vi "edittest handle delete sequence.vi"(6 "User Information":T2, 8 "error in (no error)":errorcluster, 10 "Test Sequence Id (\"\")":string, 11 "Connection Refnum":T1) -> (0 "error out":errorcluster, 3 "Connection Refnum":T1)   [LabVIEW 2011]
uses:
  server/database/Users/User Record.ctl
  Summitek EXT/ODBC/SQL Controls/Connection Refnum.ctl
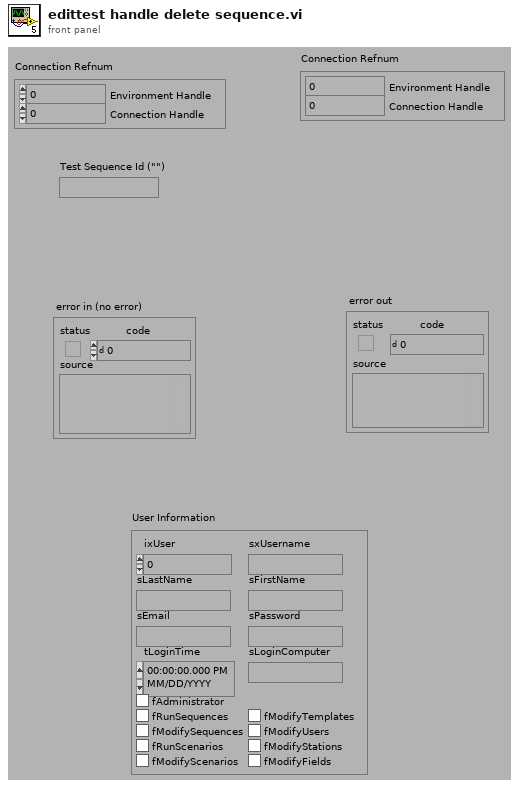
[diagram p1: front panel]
types:
  T1 = typedef "Connection Refnum.ctl" = cluster{"Environment Handle":i32, "Connection Handle":i32}
  T2 = typedef "User Record.ctl" = cluster{"ixUser":i32, "sxUsername":string, "sLastName":string, "sFirstName":string, "sEmail":string, "sPassword":string, "tLoginTime":timestamp, "sLoginComputer":string, "fAdministrator":bool, "fRunSequences":bool, "fModifySequences":bool, "fRunScenarios":bool, "fModifyScenarios":bool, "fModifyTemplates":bool, "fModifyUsers":bool, "fModifyStations":bool, "fModifyFields":bool}
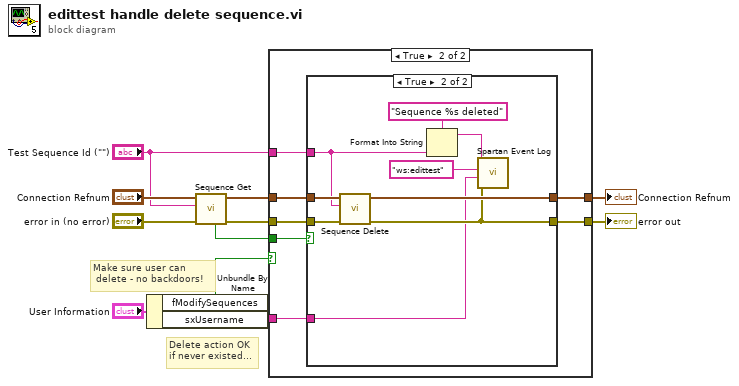
[diagram p0: block diagram]
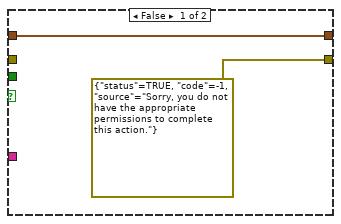
[diagram p2: hidden frame]
diagram:
  # "Delete action OK\nif never existed..."
  # "Make sure user can\n delete - no backdoors!"
  n1 = Unbundle By Name("User Information") -> ("fModifySequences"=w2:bool, "sxUsername"=w3:string)
  n2 = call "Sequence Get.vi"("error in (no error)"="error in (no error)", "sxSequenceId (\"\")"="Test Sequence Id (\"\")", "Connection Refnum"="Connection Refnum") -> ("error out"=w9:errorcluster, "Connection Refnum"=w7:T1, "Data Present"=w1:bool)  [unwired: 6 out]
  n3 = case shown="True" w2 {
    tunnel: [w13 w20] -> w11
    tunnel: [errorcluster {"status"=TRUE, "code"=-1, "source"="Sorry, you do not have the appropriate permissions to complete this action."} ("error out") w19] -> w10
    tunnel: w9 -> [_ w18]
    tunnel: w7 -> [w13 w17]
    tunnel: w3 -> [_ w15]
    tunnel: "Test Sequence Id (\"\")" -> [_ w16]
    tunnel: w1 -> [_ w14]
    frame False {
    }
    frame True {
      n4 = case shown="True" w14 {
        tunnel: [w22 w28] -> w20
        tunnel: [w21 w27] -> w19
        tunnel: w18 -> [w21 w26]
        tunnel: w17 -> [w22 w25]
        tunnel: w16 -> [_ w24]
        tunnel: w15 -> [_ w23]
        frame False {
          # "No record to delete - move on..."
        }
        frame True {
          n5 = call "Sequence Delete.vi"("error in (no error)"=w26, "Sequence ID"=w24, "Connection Refnum"=w25) -> ("error out"=w27:errorcluster, "Connection Refnum"=w28:T1)  [unwired: 7 out]
          n6 = Format Into String(format string="Sequence %s deleted" ("message (\"\")"), w24) -> (resulting string=w30:string)  [unwired: 2 in, 1 out]
          n7 = call "Spartan Event Log.vi"("error in (no error)"=w27, "username (\"\")"=w23, "module (\"\")"="ws:edittest", "message (\"\")"=w30) -> ()  [unwired: 4 in, 1 out]
        }
      }
    }
  }
  "error out" <- w10
  "Connection Refnum" <- w11
